vi "Colour up.vi"(0 "GObjects[]":refnum<vi>[](array[refnum]), 1 "Default Colour (White)":u32(colorbox)=16448250, 2 "Defined Colour (YellowLight)":u32(colorbox)=16711615, 11 "error in (no error)":errorcluster, 13 "Don't run Recursive (run)":bool) -> (15 "error out":errorcluster)   [LabVIEW 2012, in "ColourUpStructures.lvlib"]
doc: "Colour Up all Structures in <b>GObjects[]</b> Array."
uses:
  ColourUpStructures.lvlib
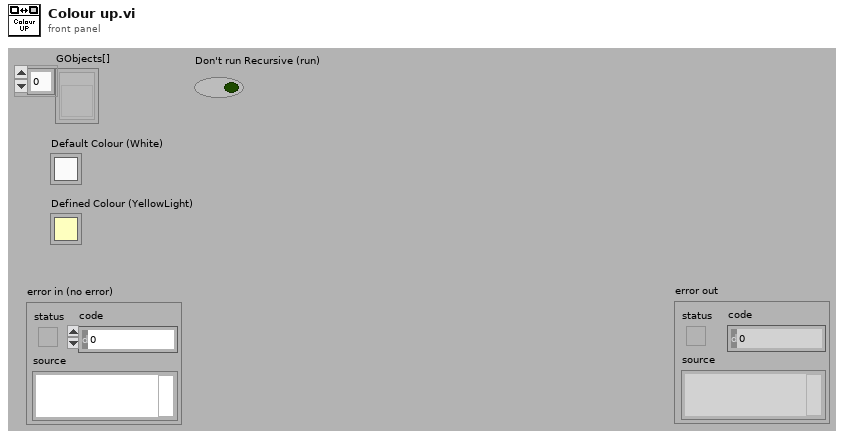
[diagram p1: front panel]
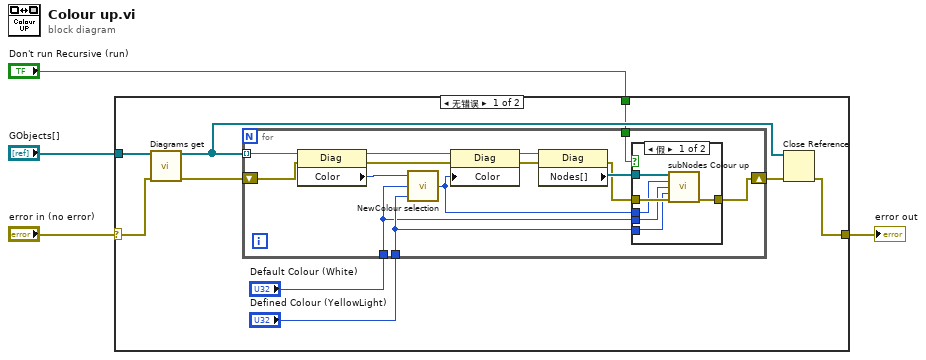
[diagram p0: block diagram]
diagram:
  n1 = case shown="无错误" "error in (no error)" {
    selector: "error in (no error)" -> [w12 w35]
    tunnel: "GObjects[]" -> [w13 _]
    tunnel: [w7 w35] -> w2
    tunnel: "Don't run Recursive (run)" -> [w5 _]
    frame No Error {
      n2 = call "Diagrams get.vi"("GObjects[]"=w13, "error in (no error)"=w12) -> ("Diagrams[]"=w9:refnum<vi>[], "error out"=w11:errorcluster)  [unwired: 12 in]
      n3 = for {
        tunnel: w9 -> [w24] mode=indexing
        shift-right: [w19] -> w10
        shift-left: w11 -> [w27]
        tunnel: "Default Colour (White)" -> [w17]
        tunnel: "Defined Colour (YellowLight)" -> [w18]
        tunnel: w5 -> [w14]
        n4 = property class="Diag"(reference=w24, error in=w27) -> (reference out=w26:refnum<vi>, error out=w25:errorcluster, "Color"=w16:u32)
        n5 = call "NewColour selection.vi"("Defined Colour"=w18, "Default Colour"=w17, "Old Color"=w16) -> ("New Colour"=w15:u32)
        n6 = property class="Diag"(reference=w26, error in=w25, "Color"=w15) -> (reference out=w22:refnum<vi>, error out=w23:errorcluster)
        n7 = property class="Diag"(reference=w22, error in=w23) -> (error out=w20:errorcluster, "Nodes[]"=w21:refnum<vi>[])  [unwired: 1 out]
        n8 = case shown="假" w14 {
          tunnel: w21 -> [w33 _]
          tunnel: w20 -> [w32 w34]
          tunnel: [w31 w34] -> w19
          tunnel: w18 -> [w30 _]
          tunnel: w17 -> [w29 _]
          tunnel: w15 -> [w28 _]
          frame False {
            n9 = call "subNodes Colour up.vi"("GObjects[]"=w33, "Parent Color"=w28, "Default Colour (White)"=w29, "Defined Colour (YellowLight)"=w30, "error in (no error)"=w32) -> ("error out"=w31:errorcluster)  [unwired: 10 in]
          }
          frame True {
          }
        }
      }
      n10 = Close Reference(reference=w9, error in (no error)=w10) -> (error out=w7:errorcluster)
    }
    frame Error {
    }
  }
  "error out" <- w2
